vi "PutBlockTable.vi"(6 "Numeric":i32, 8 "Right Block":bool, 9 "Left Block":bool, 10 "Catch Index":i16, 11 "Proc Index":i16) -> (0 "Time":i32, 1 "B":i32, 2 "A":i32, 3 "CMD":i32)   [LabVIEW 2018]
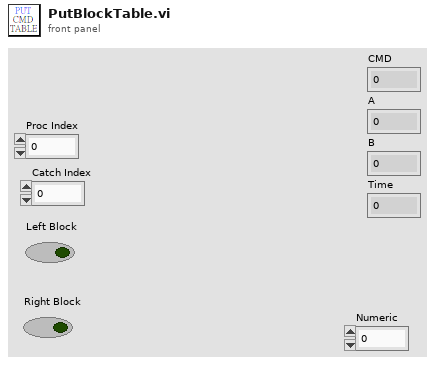
[diagram p1: front panel]
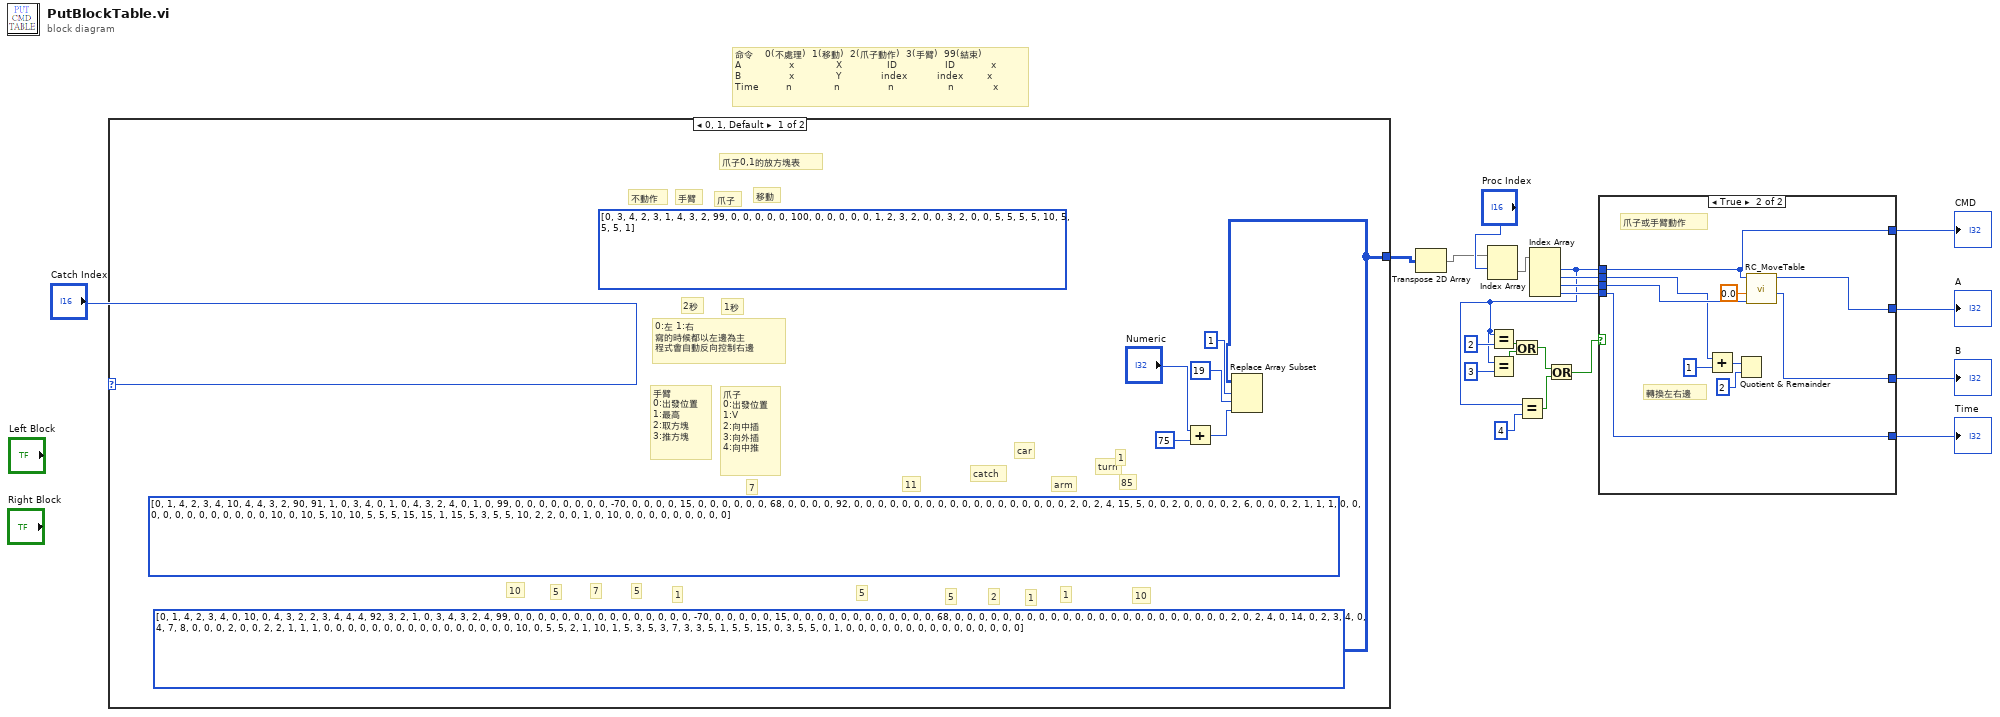
[diagram p0: block diagram]
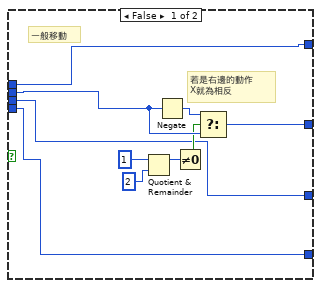
[diagram p2: hidden frame]
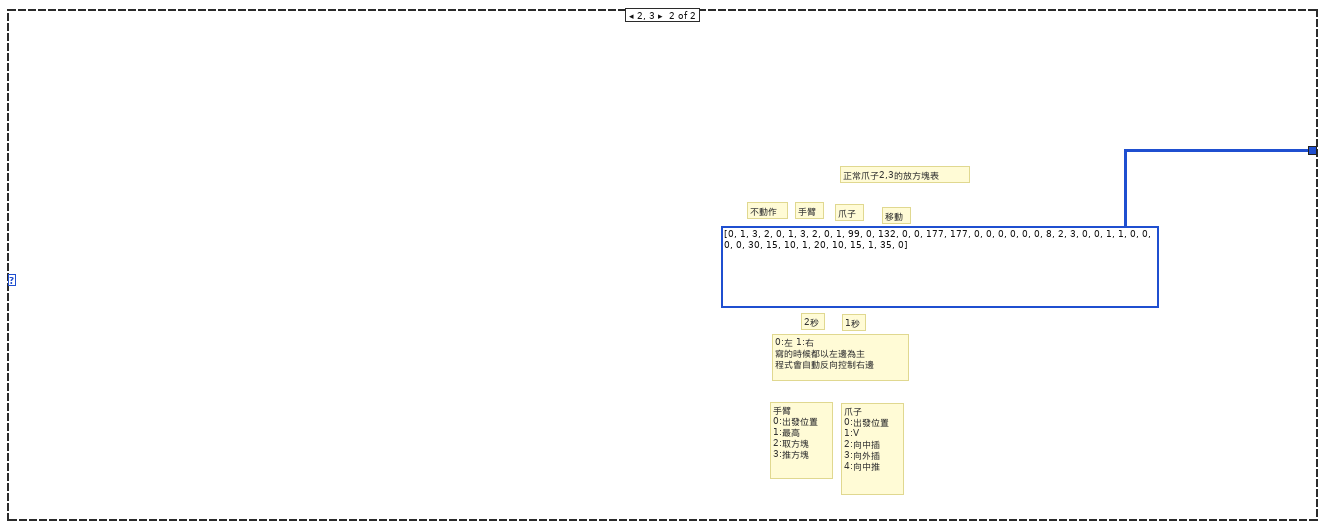
[diagram p3: hidden frame]
diagram:
  # "命令    0(不處理)  1(移動)  2(爪子動作)  3(手臂)  99(結束)\nA                x              X               ID                ID            x\nB                x              Y             index          index        x\nTime         n              n                n                  n             x"
  n1 = case shown="0, 1, Default" "Catch Index" {
    tunnel: [w22 i32[][] [[0, 1, 3, 2, 0, 1, 3, 2, 0, 1, 99], [0, 132, 0, 0, 177, 177, 0, 0, 0, 0, 0], [0, 8, 2, 3, 0, 0, 1, 1, 0, 0, 0], [0, 30, 15, 10, 1, 20, 10, 15, 1, 35, 0]]] -> w8
    frame 0, 1, Default {
      w22 = i32[][] [[0, 1, 4, 2, 3, 4, 0, 10, 0, 4, 3, 2, 2, 3, 4, 4, 4, 92, 3, 2, 1, 0, 3, 4, 3, 2, 4, 99, 0, 0, 0, 0, 0, 0, 0, 0, 0, 0, 0, 0, 0, 0], [0, -70, 0, 0, 0, 0, 0, 15, 0, 0, 0, 0, 0, 0, 0, 0, 0, 0, 0, 0, 68, 0, 0, 0, 0, 0, 0, 0, 0, 0, 0, 0, 0, 0, 0, 0, 0, 0, 0, 0, 0, 0], [0, 0, 2, 0, 2, 4, 0, 14, 0, 2, 3, 4, 0, 4, 7, 8, 0, 0, 0, 2, 0, 0, 2, 2, 1, 1, 1, 0, 0, 0, 0, 0, 0, 0, 0, 0, 0, 0, 0, 0, 0, 0], [0, 10, 0, 5, 5, 2, 1, 10, 1, 5, 3, 5, 3, 7, 3, 3, 5, 1, 5, 5, 15, 0, 3, 5, 5, 0, 1, 0, 0, 0, 0, 0, 0, 0, 0, 0, 0, 0, 0, 0, 0, 0]]
      (unwired) i32[][] [[0, 3, 4, 2, 3, 1, 4, 3, 2, 99], [0, 0, 0, 0, 0, 100, 0, 0, 0, 0], [0, 1, 2, 3, 2, 0, 0, 3, 2, 0], [0, 5, 5, 5, 5, 10, 5, 5, 5, 1]]
      (unwired) i32[][] [[0, 1, 4, 2, 3, 4, 10, 4, 4, 3, 2, 90, 91, 1, 0, 3, 4, 0, 1, 0, 4, 3, 2, 4, 0, 1, 0, 99, 0, 0, 0, 0, 0, 0, 0], [0, -70, 0, 0, 0, 0, 15, 0, 0, 0, 0, 0, 0, 68, 0, 0, 0, 0, 92, 0, 0, 0, 0, 0, 0, 0, 0, 0, 0, 0, 0, 0, 0, 0, 0], [0, 0, 2, 0, 2, 4, 15, 5, 0, 0, 2, 0, 0, 0, 0, 2, 6, 0, 0, 0, 2, 1, 1, 1, 0, 0, 0, 0, 0, 0, 0, 0, 0, 0, 0], [0, 10, 0, 10, 5, 10, 10, 5, 5, 5, 15, 15, 1, 15, 5, 3, 5, 5, 10, 2, 2, 0, 0, 1, 0, 10, 0, 0, 0, 0, 0, 0, 0, 0, 0]]
      # "3"
      # "5"
      # "turn"
      # "arm"
      # "car"
      # "catch"
      # "1"
      # "1"
      # "2"
      # "5"
      # "1"
      # "5"
      # "7"
      # "5"
      # "10"
      # "10"
      # "85"
      # "1"
      # "7"
      # "11"
      # "手臂\n0:出發位置\n1:最高\n2:取方塊\n3:推方塊"
      # "爪子\n0:出發位置\n1:V\n2:向中插\n3:向外插\n4:向中推"
      # "0:左 1:右 \n寫的時候都以左邊為主\n程式會自動反向控制右邊"
      # "爪子"
      # "移動"
      # "不動作"
      # "1秒"
      # "2秒"
      # "手臂"
      # "爪子0,1的放方塊表"
      n2 = Add(x="Numeric", y=75) -> (x+y=w24:i32)
      n3 = Replace Array Subset(array=w22, new element=w24, index (row)=1, index (col)=19 ("disabled index (col)")) -> ()  [unwired: 1 out]
    }
    frame 2, 3 {
      # "手臂\n0:出發位置\n1:最高\n2:取方塊\n3:推方塊"
      # "爪子\n0:出發位置\n1:V\n2:向中插\n3:向外插\n4:向中推"
      # "0:左 1:右 \n寫的時候都以左邊為主\n程式會自動反向控制右邊"
      # "爪子"
      # "移動"
      # "不動作"
      # "1秒"
      # "2秒"
      # "手臂"
      # "正常爪子2,3的放方塊表"
    }
  }
  n4 = Transpose 2D Array(2D array=w8) -> (transposed array=w7:i32[][])
  n5 = Index Array(array=w7, index (row)="Proc Index") -> (element=w9:i32[])  [unwired: 1 in]
  n6 = Index Array(array=w9) -> (element #1=w2:i32, element #2=w19:i32, element #3=w18:i32, element #4=w17:i32)  [unwired: 4 in]
  n7 = Equal?(x=w2, y=2) -> (x = y?=w14:bool)
  n8 = Equal?(x=w2, y=3) -> (x = y?=w4:bool)
  n9 = Or(x=w14, y=w4) -> (x .or. y?=w6:bool)
  n10 = Equal?(x=w2, y=4) -> (x = y?=w3:bool)
  n11 = Or(x=w6, y=w3) -> (x .or. y?=w5:bool)
  n12 = case shown="True" w5 {
    tunnel: w2 -> [w36 w41]
    tunnel: w19 -> [w34 w47]
    tunnel: w18 -> [w31 w48]
    tunnel: w17 -> [w30 w42]
    tunnel: [w36 w41] -> w13
    tunnel: [w32 w44] -> w12
    tunnel: [w31 w43] -> w11
    tunnel: [w30 w42] -> w10
    frame False {
      # "一般移動"
      # "若是右邊的動作\nX就為相反"
      n13 = Quotient & Remainder(x=1, y=2) -> (x-y*floor(x/y)=w37:i32)  [unwired: 1 out]
      n14 = Negate(x=w34) -> (-x=w35:i32)
      n15 = Not Equal To 0?(x=w37) -> (x != 0?=w33:bool)
      n16 = Select(t=w35, s=w33, f=w34) -> (s? t:f=w32:i32)
    }
    frame True {
      # "爪子或手臂動作"
      # "轉換左右邊"
      n17 = Add(x=w47, y=1) -> (x+y=w46:i16)
      n18 = Quotient & Remainder(x=w46, y=2) -> ()  [unwired: 2 out]
      n19 = call "RC_MoveTable.vi"("Index"=w48, "ID"=0.0, "CMD"=w41) -> ("Value"=w43:i32, "RC ID"=w44:i32)  [unwired: 6 in]
    }
  }
  "CMD" <- w13
  "A" <- w12
  "B" <- w11
  "Time" <- w10
